vi "AlliGator Build Phasor Calibration Series.vi"(8 "Error In":errorcluster, 9 "Calibration Lifetime":dbl[unit]=1e-09, 10 "Phasor Frequency":dbl[unit]=80000000.0, 11 "Uncalibrated Phasor Series":T2[](array[typedef])) -> (0 "Error Out":errorcluster, 3 "Phasor Reference Series":T1={"m Array"=[], "phi Array"=[], "Phasor Frequency"=80000000.0, "Calibration Lifetime"=1e-09})   [LabVIEW 2021, in "AlliGator Phasor Calibration.lvlib"]
doc: "Packages the provided <B>Uncalibrated Phasor Series</b> as a <B>Phasor Reference Series</B>."
uses:
  AlliGator Phasor Calibration.lvlib
  Phasor/Phasor (g, s).ctl
  Phasor/Phasor Reference Series.ctl
  Phasor/Phasor.lvlib
  Utilities/Utilities.lvlib
panel:
  # "see the AlliGator License on the block diagram (Ctrl+E or Window:Show Block Diagram)"
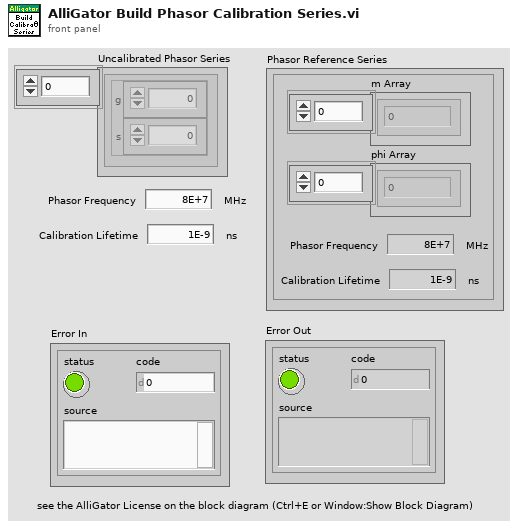
[diagram p1: front panel]
types:
  T1 = typedef "Phasor.lvlib/Phasor Reference Series.ctl" = cluster{"m Array":dbl[], "phi Array":dbl[], "Phasor Frequency":dbl[unit], "Calibration Lifetime":dbl[unit]}
  T2 = typedef "Phasor.lvlib/Phasor (g, s).ctl" = cluster{"g":dbl, "s":dbl}
  T3 = typedef "Phasor.lvlib/Phasor (m, phi).ctl" = cluster{"m":dbl, "phi":dbl}
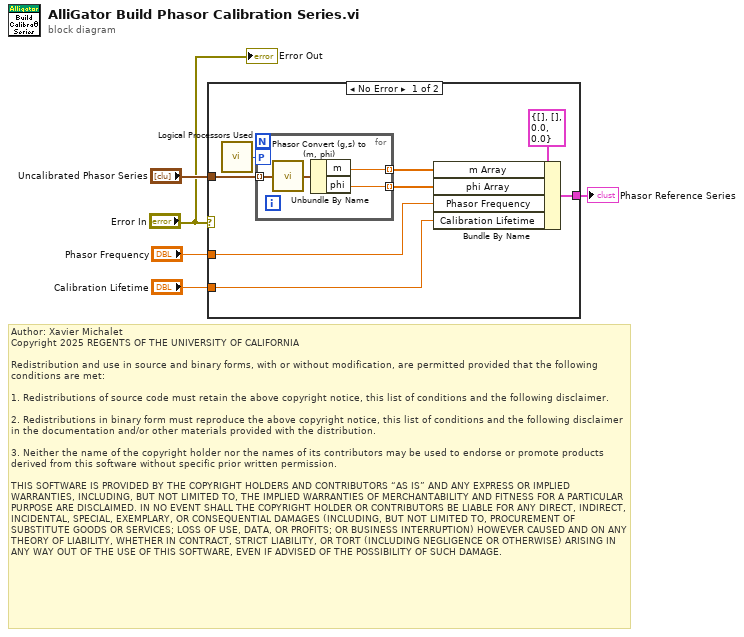
[diagram p0: block diagram]
diagram:
  # "Author: Xavier Michalet\nCopyright 2025 REGENTS OF THE UNIVERSITY OF CALIFORNIA\n\nRedistribution and use in source and binary forms, with or without modification, are permitted provided that the following conditions are met:\n\n1. Redistributions of source code must retain the above copyright notice, this list of conditions and the following disclaimer.\n\n2. Redistributions in binary form must reproduce the above copyright notice, this list of conditions and the following disclaimer in the documentation and/or other materials provided with the distribution.\n\n3. Neither the name of the copyright holder nor the names of its contributors may be used to endorse or promote products derived from this software without specific prior written permission.\n\nTHIS SOFTWARE IS PROVIDED BY THE COPYRIGHT HOLDERS AND CONTRIBUTORS “AS IS” AND ANY EXPRESS OR IMPLIED WARRANTIES, INCLUDING, BUT NOT LIMITED TO, THE IMPLIED WARRANTIES OF MERCHANTABILITY AND FITNESS FOR A PARTICULAR PURPOSE ARE DISCLAIMED. IN NO EVENT SHALL THE COPYRIGHT HOLDER OR CONTRIBUTORS BE LIABLE FOR ANY DIRECT, INDIRECT, INCIDENTAL, SPECIAL, EXEMPLARY, OR CONSEQUENTIAL DAMAGES (INCLUDING, BUT NOT LIMITED TO, PROCUREMENT OF SUBSTITUTE GOODS OR SERVICES; LOSS OF USE, DATA, OR PROFITS; OR BUSINESS INTERRUPTION) HOWEVER CAUSED AND ON ANY THEORY OF LIABILITY, WHETHER IN CONTRACT, STRICT LIABILITY, OR TORT (INCLUDING NEGLIGENCE OR OTHERWISE) ARISING IN ANY WAY OUT OF THE USE OF THIS SOFTWARE, EVEN IF ADVISED OF THE POSSIBILITY OF SUCH DAMAGE."
  n1 = case shown="No Error" "Error In" {
    tunnel: "Phasor Frequency" -> [w12 _]
    tunnel: "Calibration Lifetime" -> [w11 _]
    tunnel: [w10 _] -> w3
    tunnel: "Uncalibrated Phasor Series" -> [w9 _]
    frame No Error {
      n2 = call "Logical Processors Used.vi"() -> ("# Logical Processor Used"=w6:i32)  [unwired: 6 in]
      n3 = for {
        tunnel: w9 -> [w17] mode=indexing
        tunnel: [w16] -> w8 mode=indexing
        tunnel: [w15] -> w7 mode=indexing
        workers-P: w6 -> [_]
        n4 = call "Phasor Convert (g,s) to (m, phi).vi"("Phasor (g, s)"=w17) -> ("Phasor (m, phi)"=w14:T3)  [unwired: 8 in]
        n5 = Unbundle By Name(w14) -> ("m"=w16:dbl, "phi"=w15:dbl)
      }
      n6 = Bundle By Name(cluster=T1 {"m Array"=[], "phi Array"=[], "Phasor Frequency"=0.0, "Calibration Lifetime"=0.0} ("Phasor Reference Plot"), "m Array"=w8, "phi Array"=w7, "Phasor Frequency"=w12, "Calibration Lifetime"=w11) -> (w10:T1)
    }
    frame Error {
    }
  }
  "Phasor Reference Series" <- w3
  "Error Out" <- "Error In"
